vi "Channel Specification.vi"(8 "error in":errorcluster, 11 "Node Ptr":T1 format="%.0x") -> (0 "error out":errorcluster)   [LabVIEW 2020, in "Ballard ARINC 429 System Explorer.lvlib" / "Implementation.lvlib"]
uses:
  Implementation.lvlib
  <vilib>/NI VeriStand/Custom Device API/Custom Device Item Ref.ctl
  <vilib>/NI VeriStand/Custom Device API/Custom Device API.lvlib
  Scripting/Ballard ARINC 429 Scripting.lvlib
panel:
  out "Channel Settings":string[][](table)=[["Type", "Input"], ["Units", ""], ["Default Value", "3.000000"], ["Faultable", "No"], ["Scalable", "No"]]
  in  "Default Value":dbl=3.0
  in  "SHDocVw.IWebBrowser":refnum<k7>(container)
  in  "General Header":cluster{"Section Name":string}={"Section Name"="Ballard ARINC 429 - Channel Specification"}
  in  "Description":string
  out "Name":string
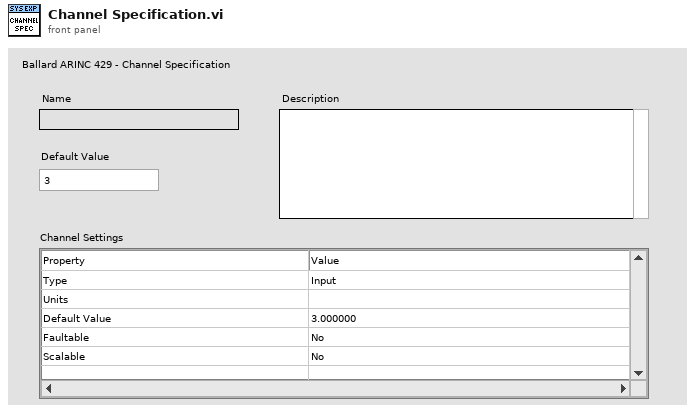
[diagram p1: front panel]
types:
  T1 = typedef "Custom Device API.lvlib/Custom Device Item Ref.ctl" = u64
  T2 = typedef "Custom Device API.lvlib/Custom Device Channel.ctl" = cluster{"Type":T3, "Units":string, "Default Value":dbl, "Faultable":bool, "Scalable":bool}
  T3 = typedef "Custom Device API.lvlib/Custom Device Channel Type.ctl" = enum16{"Input", "Output"}
  T4 = typedef "Custom Device API.lvlib/Custom Device Item Info.ctl" = cluster{"Name":string, "Is Channel":bool, "GUID":string, "Is Waveform":bool}
  T5 = typedef "Custom Device API.lvlib/Custom Device Commands.ctl" = enum16{"Default", "Item renamed", "Shutdown", "Dynamic button pressed"}
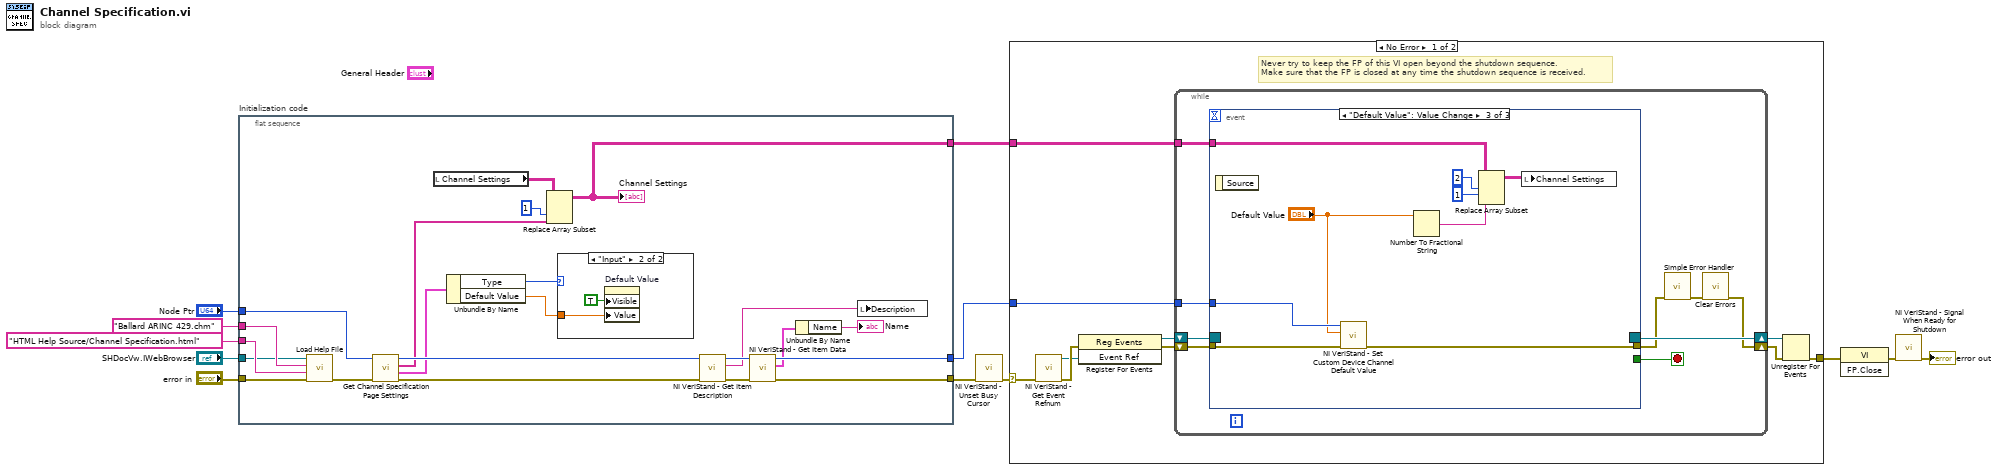
[diagram p0: block diagram]
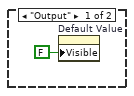
[diagram p2: hidden frame]
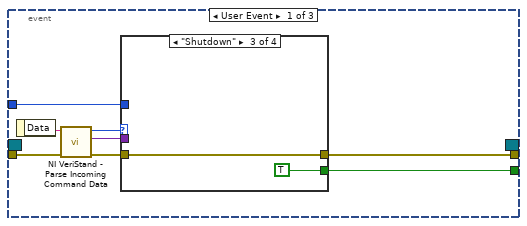
[diagram p3: hidden frame]
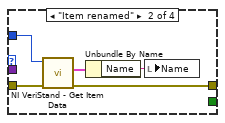
[diagram p5: hidden frame]
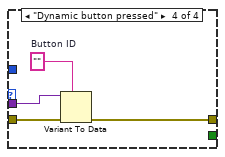
[diagram p6: hidden frame]
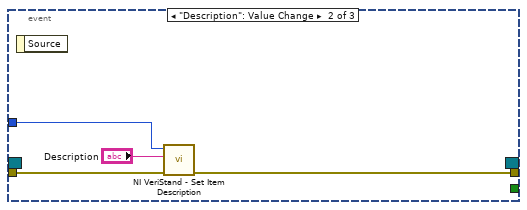
[diagram p7: hidden frame]
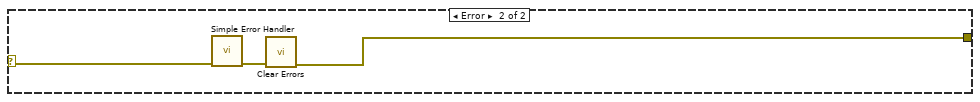
[diagram p8: hidden frame]
diagram:
  n1 = flat-sequence "Initialization code" {
    tunnel: "error in" -> [w28]
    tunnel: "Node Ptr" -> [w20]
    tunnel: [w30] -> w8
    tunnel: [w34] -> w5
    tunnel: "SHDocVw.IWebBrowser" -> [w25]
    tunnel: "HTML Help Source/Channel Specification.html" ("CD_CHM_Section") -> [w27]
    tunnel: "Ballard ARINC 429.chm" ("CD_CHM_FileName") -> [w26]
    tunnel: [w13] -> w1
    frame #0 {
      n2 = call "Load Help File.vi"("error in (no error)"=w28, "HTML File to Load"=w27, "Main CHM File"=w26, "Browser"=w25) -> ("error out"=w18:errorcluster)  [unwired: 7 in]
      n3 = call "Get Channel Specification Page Settings.vi"("error in"=w18, "parameter ref"=w20) -> ("error out"=w17:errorcluster, "Channel"=w15:T2, "Channel Settings"=w14:string[], "parameter ref out"=w19:T1)  [unwired: 6 in]
      n4 = local read "Channel Settings"() -> (w23:string[][])
      n5 = Unbundle By Name(w15) -> ("Type"=w21:T3, "Default Value"=w16:dbl)
      n6 = Replace Array Subset(array=w23, new element=w14, index (col)=1 ("disabled index (col)")) -> (w13:string[][])  [unwired: 1 in]
      "Channel Settings" <- w13
      n7 = case shown="\"Input\"" w21 {
        tunnel: w16 -> [_ w37]
        frame "Output" {
          n8 = property on="Default Value" class="DigNum (strict)"("Visible"=FALSE) -> ()  [unwired: 2 in, 2 out]
        }
        frame "Input" {
          n9 = property on="Default Value" class="DigNum (strict)"("Visible"=TRUE, "Value"=w37) -> ()  [unwired: 2 in, 2 out]
        }
      }
      n10 = call <vilib>:"NI VeriStand - Get Item Description.vi"("error in (no error)"=w17, "Item Ref in"=w19) -> ("error out"=w32:errorcluster, "Description"=w29:string, "Item Ref out"=w33:T1)  [unwired: 7 out]
      n11 = call <vilib>:"NI VeriStand - Get Item Data.vi"("error in (no error)"=w32, "Item Ref in"=w33) -> ("error out"=w30:errorcluster, "Item Info"=w31:T4, "Item Ref out"=w34:T1)  [unwired: 7 out]
      n12 = Unbundle By Name(w31) -> ("Name"=→"Name":string)
      n13 = local write "Description"(w29) -> ()
    }
  }
  n14 = call <vilib>:"NI VeriStand - Unset Busy Cursor.vi"("error in (no error)"=w8) -> ("error out"=w7:errorcluster)  [unwired: 10 out]
  n15 = case shown="No Error" w7 {
    selector: w7 -> [w39 w92]
    tunnel: [w44 w90] -> w12
    tunnel: w5 -> [w40 _]
    tunnel: w1 -> [w38 _]
    frame No Error {
      # "Never try to keep the FP of this VI open beyond the shutdown sequence.\nMake sure that the FP is closed at any time the shutdown sequence is received."
      n16 = call <vilib>:"NI VeriStand - Get Event Refnum.vi"("error in (no error)"=w39) -> ("error out"=w47:errorcluster, "Event Ref"=w43:refnum<user-event>)  [unwired: 9 out]
      n17 = register-events(error in=w47, w43) -> (reference out=w41:refnum<event-registration>, error out=w42:errorcluster)  [unwired: 1 in]
      n18 = while {
        tunnel: w40 -> [w52]
        shift-right: [w49] -> w45
        shift-left: w42 -> [w55]
        shift-right: [w56] -> w46
        shift-left: w41 -> [w54]
        tunnel: w38 -> [w48]
        stop <- w53 stop-if-true
        n19 = event shown="[2] \"Default Value\": Value Change" {
          selector: w54 -> [_ _ _]
          dyn-events: [_ _ _] -> w56
          timeout: _ -> [_ _ _]
          tunnel: w55 -> [w64 w79 w88]
          tunnel: [w60 _ _] -> w53
          tunnel: [w59 w78 w87] -> w51
          tunnel: w52 -> [w58 w80 w89]
          tunnel: w48 -> [_ _ w86]
          event User Event {
            n20 = event-data() -> ("Data"=w63:string)  [unwired: 1 out]
            n21 = call <vilib>:"NI VeriStand - Parse Incoming Command Data.vi"("error in (no error)"=w64, "Incoming data"=w63) -> ("error out"=w62:errorcluster, "Outgoing data"=w57:variant, "Action"=w61:T5)  [unwired: 7 out]
            n22 = case shown="\"Shutdown\"" w61 {
              tunnel: w62 -> [w65 w70 w71 w76]
              tunnel: [_ _ TRUE _] -> w60
              tunnel: [w65 w67 w71 w73] -> w59
              tunnel: w58 -> [_ w69 _ _]
              tunnel: w57 -> [_ _ _ w75]
              frame "Default", Default {
              }
              frame "Item renamed" {
                n23 = call <vilib>:"NI VeriStand - Get Item Data.vi"("error in (no error)"=w70, "Item Ref in"=w69) -> ("error out"=w67:errorcluster, "Item Info"=w68:T4)  [unwired: 8 out]
                n24 = Unbundle By Name(w68) -> ("Name"=w66:string)
                n25 = local write "Name"(w66) -> ()
              }
              frame "Shutdown" {
              }
              frame "Dynamic button pressed" {
                w74 = ""  # Button ID
                n26 = Variant To Data(error in=w76, type=w74, Variant=w75) -> (error out=w73:errorcluster)  [unwired: 1 out]
              }
            }
          }
          event "Description": Value Change {
            n27 = event-data() -> ()  [unwired: 2 out]
            n28 = call <vilib>:"NI VeriStand - Set Item Description.vi"("error in (no error)"=w79, "Description"="Description", "Item Ref in"=w80) -> ("error out"=w78:errorcluster)  [unwired: 8 out]
          }
          event "Default Value": Value Change {
            n29 = event-data() -> ()  [unwired: 2 out]
            n30 = call <vilib>:"NI VeriStand - Set Custom Device Channel Default Value.vi"("error in (no error)"=w88, "Default Value"="Default Value", "Channel Ref in"=w89) -> ("error out"=w87:errorcluster)  [unwired: 7 in, 1 out]
            n31 = Number To Fractional String(number="Default Value") -> (F-format string=w82:string)  [unwired: 3 in]
            n32 = Replace Array Subset(array=w86, new element=w82, index (row)=2, index (col)=1 ("disabled index (col)")) -> (w85:string[][])
            n33 = local write "Channel Settings"(w85) -> ()
          }
        }
        n34 = call <vilib>:"Simple Error Handler.vi"("error in (no error)"=w51) -> ("error out"=w50:errorcluster)  [unwired: 1 in, 7 out]
        n35 = call <vilib>:"Clear Errors.vi"("error in (no error)"=w50) -> ("error out"=w49:errorcluster)  [unwired: 1 in, 5 out]
      }
      n36 = Unregister For Events(event registration refnum=w46, error in=w45) -> (error out=w44:errorcluster)
    }
    frame Error {
      n37 = call <vilib>:"Simple Error Handler.vi"("error in (no error)"=w92) -> ("error out"=w91:errorcluster)  [unwired: 1 in, 7 out]
      n38 = call <vilib>:"Clear Errors.vi"("error in (no error)"=w91) -> ("error out"=w90:errorcluster)  [unwired: 1 in, 5 out]
    }
  }
  n39 = invoke class="VI" method="FP.Close"(error in=w12) -> (error out=w11:errorcluster)  [unwired: 2 in, 2 out]
  n40 = call <vilib>:"NI VeriStand - Signal When Ready for Shutdown.vi"("error in (no error)"=w11) -> ("error out"=→"error out":errorcluster)  [unwired: 10 out]
